vi "test negative timestamp.vi"(8 "error in (no error)":errorcluster, 11 "TestCase in":refnum<class "Timestamp Tests.lvclass">) -> (0 "error out":errorcluster, 3 "TestCase out":refnum<class "Timestamp Tests.lvclass">)   [LabVIEW 2020]
uses:
  Timestamp Tests.lvclass
  <vilib>/Utility/file.llb/Application Directory.vi
  <vilib>/Utility/libraryn.llb/Check if File or Folder Exists.vi
  <vilib>/addons/_JKI Toolkits/VI Tester/TestCase.llb/TestCase.lvclass
  C:/Program Files (x86)/National Instruments/LabVIEW 2020/vi.lib/addons/_JKI Toolkits/VI Tester/TestCase.llb/TestCase.lvclass
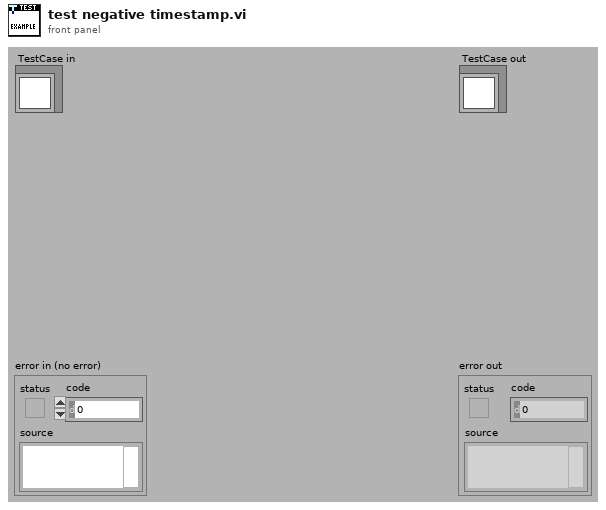
[diagram p1: front panel]
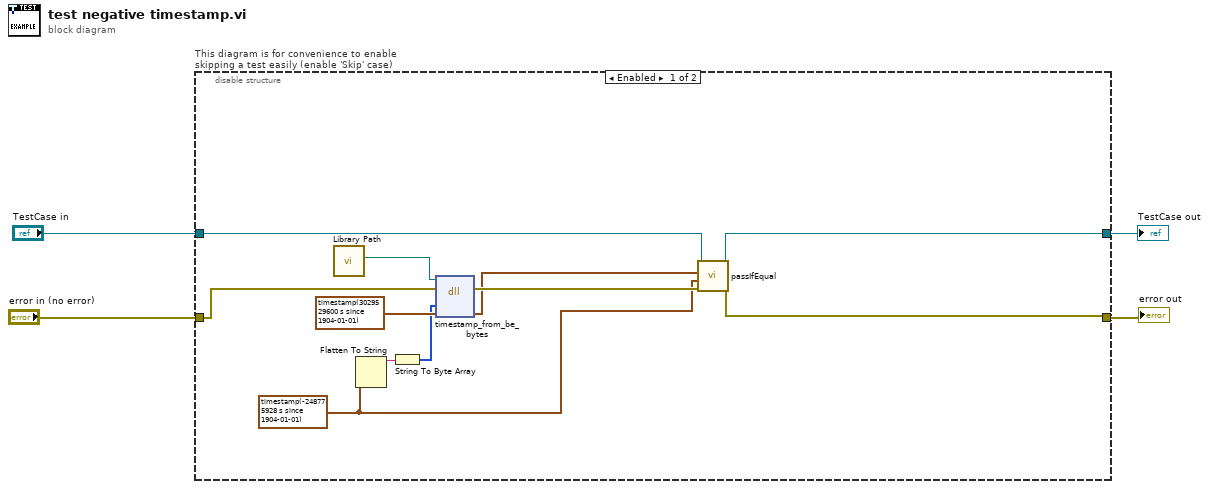
[diagram p0: block diagram]
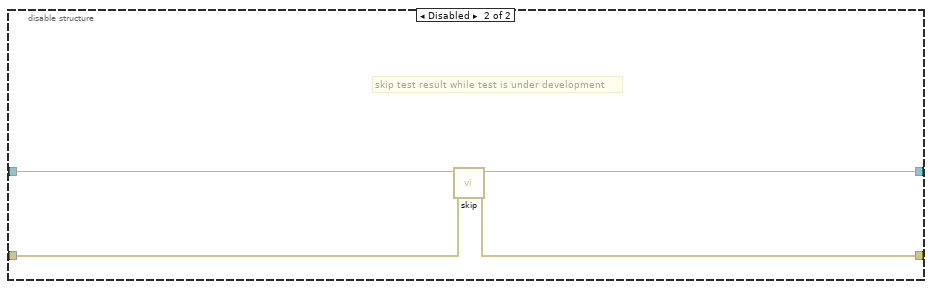
[diagram p2: hidden frame]
diagram:
  n1 = disable-structure "This diagram is for convenience to enable skipping a test easily (enable 'Skip' case)" shown="Enabled" {
    disable-tunnel: "TestCase in" -> [w15 w19]
    disable-tunnel: [w14 w17] -> w1
    disable-tunnel: [w13 w18] -> w3
    disable-tunnel: "error in (no error)" -> [w12 w16]
    frame Enabled {
      w8 = timestamp(-248775927.976 s since 1904-01-01) ("Time Stamp")
      n2 = call "Library Path.vi"() -> ("Library Path"=w5:path)  [unwired: 11 in]
      n3 = Flatten To String(anything=w8) -> (data string=w7:string)  [unwired: 3 in, 2 out]
      n4 = String To Byte Array(string=w7) -> (unsigned byte array=w6:u8[])
      n5 = dll-call lib="C:/Users/JamesMcNally/Documents/RustInterop/Rust-LabVIEW-Interop/target/debug/labview_test_library.dll" fn="timestamp_from_be_bytes"(path in=w5, error in=w12, "bytes"=w6, "timestamp"=timestamp(3029529600 s since 1904-01-01) ("Time Stamp")) -> (error out=w11:errorcluster, "timestamp"=w9:timestamp)  [unwired: 3 in, 1 out]
      n6 = call-dynamic "passIfEqual.vi"("error in (no error)"=w11, "y"=w8, "x"=w9, "TestCase in"=w15) -> ("error out"=w13:errorcluster, "TestCase out"=w14:refnum<class "Timestamp Tests.lvclass">)  [unwired: 6 in]
    }
    frame Disabled {
      # "skip test result while test is under development"
      n7 = call <vilib>:"skip.vi"("error in (no error)"=w16, "TestCase in"=w19) -> ("error out"=w18:errorcluster, "TestCase out"=w17:refnum<class "Timestamp Tests.lvclass">)  [unwired: 8 in]
    }
  }
  "error out" <- w3
  "TestCase out" <- w1
